vi "process.vi"(8 "error in":errorcluster, 9 "results data":T1, 10 "parameters data":T1, 11 "module in":refnum<class "Shared Memory Runtime.lvclass">) -> (0 "error out":errorcluster, 1 "results data out":T1, 2 "parameter data out":T1, 3 "module out":refnum<class "Shared Memory Runtime.lvclass">)   [LabVIEW 2013, in "shared memory runtime.lvclass"]
doc: "Provides an interface for information processing by a module at runtime. While this interface performs no operations, a child should provide an override which may process data in any manner necessary."
uses:
  Shared Memory Runtime.lvclass
  <vilib>/NI/Tag Bus/table/data table.ctl
  <vilib>/NI/Tag Bus Module Framework/channel/channel classification.ctl
  <vilib>/NI/Tag Bus Module Framework/channel/TBM channel.lvclass
  <vilib>/NI/Tag Bus/table/data table.lvlib
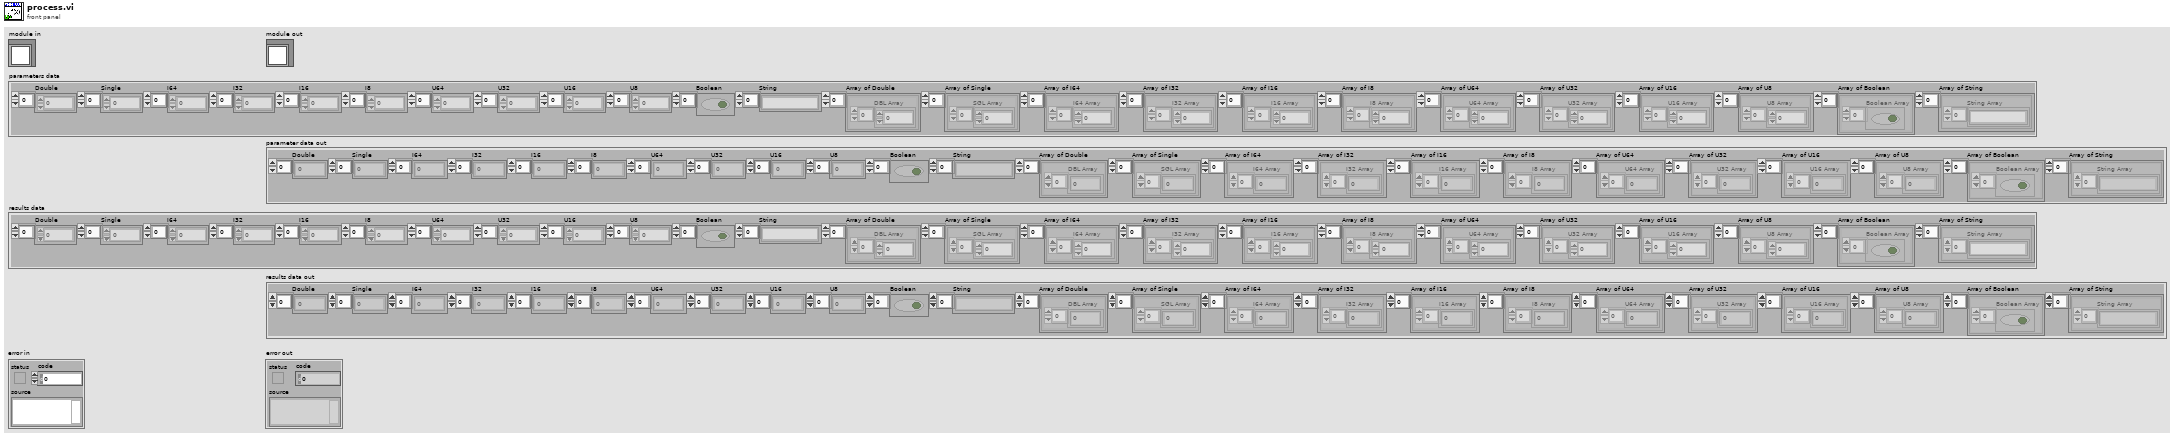
[diagram p1: front panel]
types:
  T1 = typedef "tag bus.lvlib/data table.lvlib/data table.ctl" = cluster{"Double":dbl[], "Single":sgl[], "I64":i64[], "I32":i32[], "I16":i16[], "I8":i8[], "U64":u64[], "U32":u32[], "U16":u16[], "U8":u8[], "Boolean":bool[], "String":string[], "Array of Double":cluster{"DBL Array":dbl[]}[], "Array of Single":cluster{"SGL Array":sgl[]}[], "Array of I64":cluster{"I64 Array":i64[]}[], "Array of I32":cluster{"I32 Array":i32[]}[], "Array of I16":cluster{"I16 Array":i16[]}[], "Array of I8":cluster{"I8 Array":i8[]}[], "Array of U64":cluster{"U64 Array":u64[]}[], "Array of U32":cluster{"U32 Array":u32[]}[], "Array of U16":cluster{"U16 Array":u16[]}[], "Array of U8":cluster{"U8 Array":u8[]}[], "Array of Boolean":cluster{"Boolean Array":bool[]}[], "Array of String":cluster{"String Array":string[]}[]}
  T2 = typedef "TBM channel.lvclass/channel classification.ctl" = enum16{"input data", "output data", "processing parameter", "processing result"}
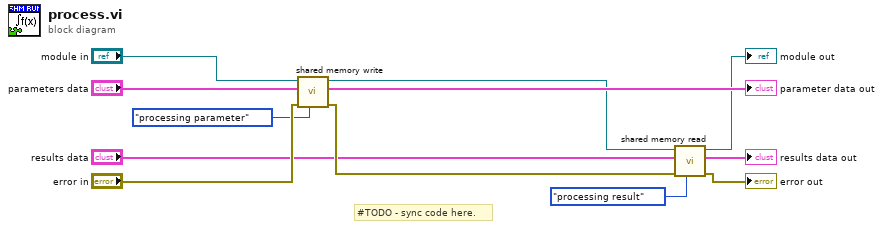
[diagram p0: block diagram]
diagram:
  # "#TODO - sync code here."
  n1 = call "shared memory write.vi"("channel classification"=channel_classification."processing parameter", "error in"="error in", "data table"="parameters data", "module in"="module in") -> ("error out"=w11:errorcluster, "data table out"=→"parameter data out":T1, "module out"=w1:refnum<class "Shared Memory Runtime.lvclass">)  [unwired: 5 in]
  n2 = call "shared memory read.vi"("channel classification"=channel_classification."processing result", "error in"=w11, "data table"="results data", "module in"=w1) -> ("error out"=→"error out":errorcluster, "data table out"=→"results data out":T1, "module out"=→"module out":refnum<class "Shared Memory Runtime.lvclass">)  [unwired: 5 in]
